vi "Display Error.vi"(8 "error in (no error)":errorcluster, 10 "Error message":string, 11 "Monitor-Pulse in":refnum<class "Application Controller.lvclass">) -> (0 "error out":errorcluster, 3 "Monitor-Pulse out":refnum<class "Application Controller.lvclass">)   [LabVIEW 2016, in "Application Controller.lvclass"]
uses:
  Application Controller.lvclass
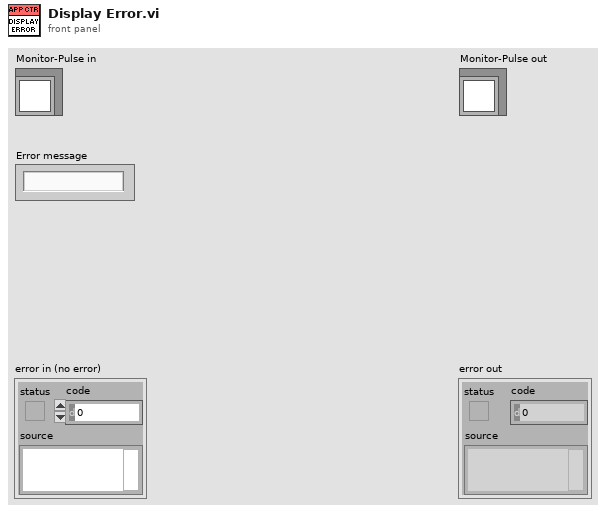
[diagram p1: front panel]
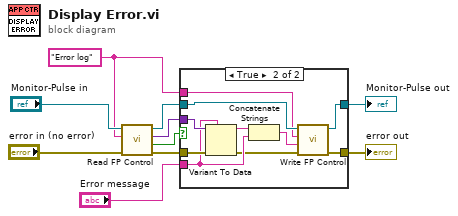
[diagram p0: block diagram]
diagram:
  w5 = "Error log" ("Control Name")
  n1 = call-dynamic "Read FP Control.vi"("error in (no error)"="error in (no error)", "Control Name"=w5, "Measure Object in"="Monitor-Pulse in") -> ("error out"=w8:errorcluster, "Present"=w1:bool, "Control Value"=w9:variant, "Measure Object out"=w6:refnum<class "Application Controller.lvclass">)  [unwired: 5 in]
  n2 = case shown="True" w1 {
    tunnel: w9 -> [_ w22]
    tunnel: w8 -> [w12 w21]
    tunnel: "Error message" -> [_ w19]
    tunnel: w6 -> [w11 w18]
    tunnel: w5 -> [_ w17]
    tunnel: [w12 w14] -> w4
    tunnel: [w11 w13] -> w3
    frame False {
    }
    frame True {
      n3 = Variant To Data(error in=w21, type=w19, Variant=w22) -> (data=w20:string, error out=w15:errorcluster)
      n4 = Concatenate Strings(w20, w19) -> (w16:string)
      n5 = call-dynamic "Write FP Control.vi"("error in (no error)"=w15, "Control Value"=w16, "Control Name"=w17, "Measure Object in"=w18) -> ("error out"=w14:errorcluster, "Measure Object out"=w13:refnum<class "Application Controller.lvclass">)  [unwired: 6 in]
    }
  }
  "error out" <- w4
  "Monitor-Pulse out" <- w3
